vi "定时触发器.vi"(9 "绝对定时忽略0帧? (T)":bool=TRUE, 10 "定时配置":T1={"定时模式"=enum."绝对时间", "单位"=enum."年", "间隔"=1, "目标时刻"=timestamp(0 s since 1904-01-01)} {"间隔" min=1}, 11 "定时器结构名":string="L229074972") -> ()   [LabVIEW 2017]
doc: "可重入的定时触发源, 相对定时和绝对定时. \n\n绝对定时 在运行启动或重新配置之后,可按需求设定是否忽略0帧触发;\n相对定时 在运行启动时重新配置之后,强制执行0帧触发."
uses:
  <vilib>/Platform/TimedLoop/XDataNode/timing_clust.ctl
  <vilib>/Platform/TimedLoop/XDataNode/nitl_modes.ctl
  <vilib>/Platform/TimedLoop/XDataNode/wakeup.ctl
  <vilib>/Platform/TimedLoop/XDataNode/XDataNode.xnode
  <vilib>/Platform/TimedLoop/XDataNode/XDNodeRunTimeDep.lvlib
panel:
  in  "重启定时":bool
  in  "结构名":string="L229074972"
  out "上次触发":timestamp
  # "用法:\n1. 使用异步调用\n2. 改变输入, 调用定时结构停止函数, 实现重启并应用新的定时配置\n\n注意:\n此VI中, 首次启动或重新配置定时循环时不触发值改变事件"
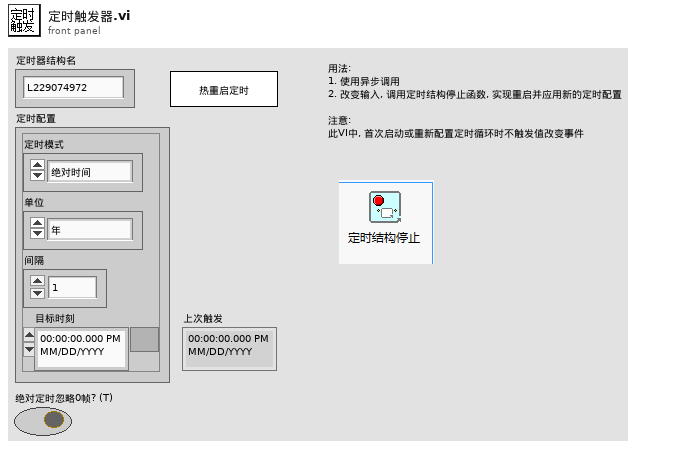
[diagram p1: front panel]
types:
  T1 = typedef "簇-定时配置.ctl" = cluster{"定时模式":enum16{"绝对时间", "相对时间"}, "单位":enum16{"年", "月", "日", "时", "分"}, "间隔":u8, "目标时刻":timestamp}
  T2 = typedef "XDNodeRunTimeDep.lvlib/timing_clust.ctl" = cluster{"Expected End [f-1]":u64, "Actual End [f-1]":u64, "Finished Late? [f-1]":bool, "Expected End [i-1]":u64, "Actual End [i-1]":u64, "Finished Late? [i-1]":bool, "Expected Start [i]":u64, "Actual Start [i]":u64, "Expected Start [f]":u64, "Actual Start [f]":u64, "Source Name":string, "Structure Name":string, "Period":i64, "Deadline":i64, "Offset":i64, "Start":i64, "Priority":i32, "Timeout":i32, "Mode":T3, "Wakeup Reason":T4, "Error":errorcluster, "Source Type":string, "Secondary Source Type":string, "Global End Time":u64, "Global Start Time":u64, "Frame Duration":u64, "Iteration Duration":u64, "Assigned CPU":i32, "I/O Scan Engine Mode":u32}
  T3 = typedef "XDNodeRunTimeDep.lvlib/nitl_modes.ctl" = enum32{"No Change", "Process missed periods, maintain original phase", "Discard missed periods, maintain original phase", "Process missed periods, ignore original phase", "Discard missed periods, ignore original phase"}
  T4 = typedef "XDNodeRunTimeDep.lvlib/wakeup.ctl" = enum32{"Normal", "Aborted", "Asynchronous wakeup", "Timing source error", "Timed loop error", "Timeout"}
  T5 = typedef "LVDateTimeRec.ctl" = cluster{"秒数的小数部分":dbl, "秒":i32, "分":i32, "时":i32, "日":i32, "月":i32, "年":i32, "天数（周）":i32, "天数（年）":i32, "DST":i32}
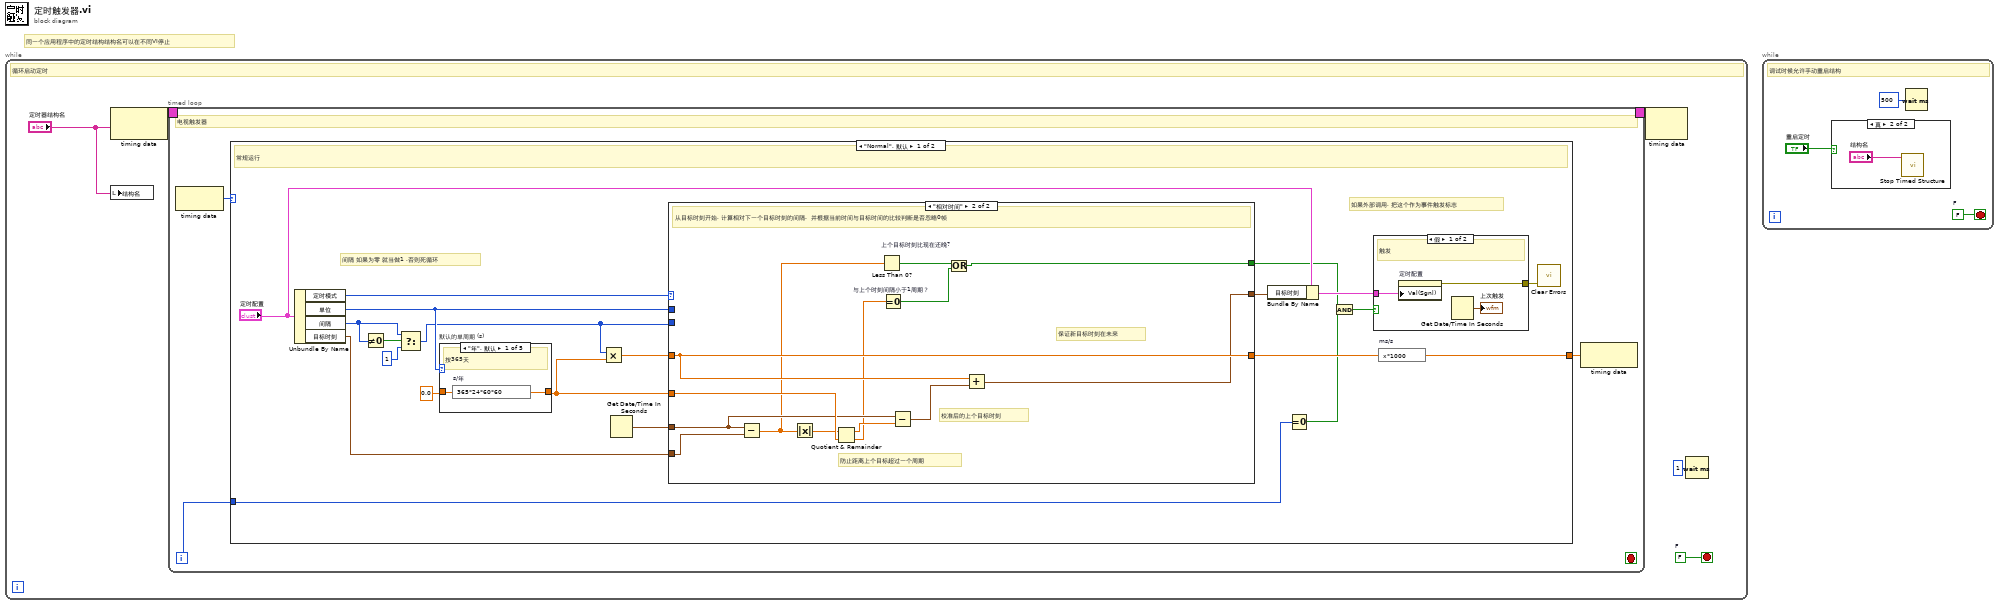
[diagram p0: block diagram]
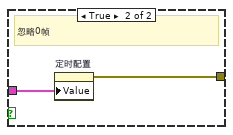
[diagram p3: hidden frame]
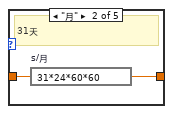
[diagram p4: hidden frame]
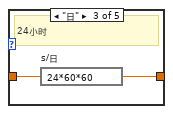
[diagram p5: hidden frame]
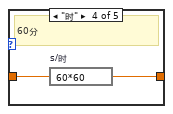
[diagram p6: hidden frame]
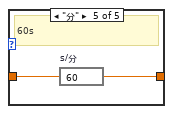
[diagram p7: hidden frame]
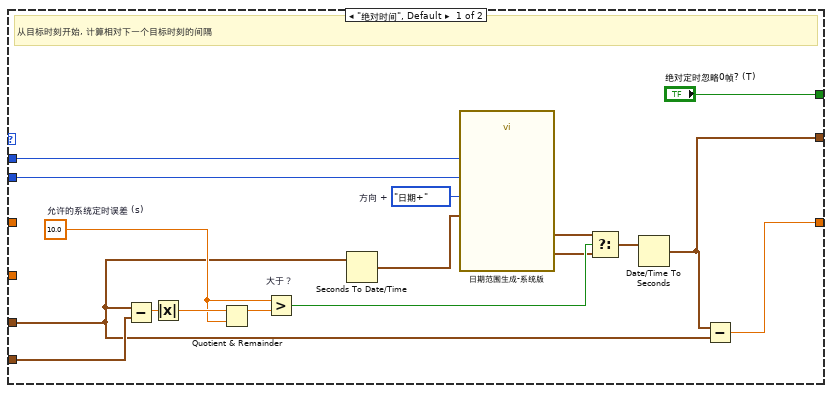
[diagram p8: hidden frame]
diagram:
  # "同一个应用程序中的定时结构结构名可以在不同VI停止"
  n1 = while {
    stop <- w3 stop-if-true
    w3 = FALSE  # F
    # "循环启动定时"
    n2 = node-c288("定时器结构名") -> (w5:T2)
    n3 = local write "结构名"("定时器结构名") -> ()
    n4 = timed-loop {
      timing: w5 -> [_]
      timing-out: [_] -> w4
      i -> [w7]
      stop <- _ stop-if-true
      # "电视触发器"
      n5 = node-c288() -> (w6:T4)  [unwired: 1 in]
      n6 = case shown="\"Normal\", 默认" w6 {
        tunnel: [w25 _] -> w8
        tunnel: w7 -> [w15 _]
        frame "Normal", Default {
          # "间隔 如果为零 就当做1 ,否则死循环"
          # "如果外部调用, 把这个作为事件触发标志"
          # "常规运行"
          n7 = Unbundle By Name("定时配置") -> ("定时模式"=w29:enum16{"绝对时间", "相对时间"}, "单位"=w28:enum16{"年", "月", "日", "时", "分"}, "间隔"=w17:u8, "目标时刻"=w24:timestamp)
          n8 = Not Equal To 0?(x=w17) -> (x != 0?=w19:bool)
          n9 = Select(t=w17, s=w19, f=u8 1 ("间隔")) -> (s? t:f=w16:u8)
          n10 = case "默认的单周期 (s)" shown="\"年\", 默认" w28 {
            tunnel: [w36 w38 w40 w42 w44] -> w9
            tunnel: 0.0 -> [w35 w37 w39 w41 w43]
            frame "年", Default {
              # "按365天"
              n11 = expression code="365*24*60*60" "s/年"(w35) -> (w36:dbl)
            }
            frame "月" {
              # "31天"
              n12 = expression code="31*24*60*60" "s/月"(w37) -> (w38:dbl)
            }
            frame "日" {
              # "24小时"
              n13 = expression code="24*60*60" "s/日"(w39) -> (w40:dbl)
            }
            frame "时" {
              # "60分"
              n14 = expression code="60*60" "s/时"(w41) -> (w42:dbl)
            }
            frame "分" {
              # "60s"
              n15 = expression code="60" "s/分"(w43) -> (w44:dbl)
            }
          }
          n16 = Multiply(x=w16, y=w9) -> (x*y=w23:dbl)
          n17 = Get Date/Time In Seconds() -> (seconds since 1Jan1904=w10:timestamp)
          n18 = case shown="\"相对时间\"" w29 {
            tunnel: w28 -> [w61 _]
            tunnel: w16 -> [w56 _]
            tunnel: [w59 w74] -> w26
            tunnel: w24 -> [w57 w69]
            tunnel: w23 -> [_ w74]
            tunnel: [w55 w73] -> w20
            tunnel: ["绝对定时忽略0帧? (T)" w64] -> w11
            tunnel: w10 -> [w45 w71]
            tunnel: w9 -> [_ w72]
            frame "绝对时间", Default {
              w47 = 10.0  # 允许的系统定时误差 (s)
              w54 = enum16{"当前", "日期+", "日期-"}."日期+"  # 方向 +
              # "从目标时刻开始, 计算相对下一个目标时刻的间隔"
              n19 = Subtract(x=w45, y=w57) -> (x-y=w58:dbl)
              n20 = Absolute Value(x=w58) -> (abs(x)=w49:dbl)
              n21 = Quotient & Remainder(x=w49, y=w47) -> (x-y*floor(x/y)=w48:dbl)  [unwired: 1 out]
              n22 = Greater? "大于？"(x=w47, y=w48) -> (0:w53:bool)
              n23 = Seconds To Date/Time(time stamp (now)=w45) -> (date time rec=w60:T5)  [unwired: 1 in]
              n24 = call "日期范围生成-系统版.vi"("单位"=w61, "方向"=w54, "变化量(1)"=w56, "日期时间记录"=w60) -> ("下限"=w51:T5, "上限"=w50:T5)  [unwired: 6 in]
              n25 = Select(t=w51, s=w53, f=w50) -> (s? t:f=w52:T5)
              n26 = Date/Time To Seconds(2:w52) -> (0:w55:timestamp)  [unwired: 1 in]
              n27 = Subtract(x=w55, y=w45) -> (x-y=w59:dbl)
            }
            frame "相对时间" {
              # "保证新目标时刻在未来"
              # "校准后的上个目标时刻"
              # "防止距离上个目标超过一个周期"
              # "从目标时刻开始, 计算相对下一个目标时刻的间隔.  并根据当前时间与目标时间的比较判断是否忽略0帧"
              n28 = Subtract(x=w71, y=w69) -> (x-y=w66:dbl)
              n29 = Absolute Value(x=w66) -> (abs(x)=w67:dbl)
              n30 = Quotient & Remainder(x=w67, y=w72) -> (x-y*floor(x/y)=w70:dbl, floor(x/y)=w63:dbl)
              n31 = Less Than 0? "上个目标时刻比现在还晚?"(x=w66) -> (x < 0?=w65:bool)
              n32 = Equal To 0? "与上个时刻间隔小于1周期？"(x=w63) -> (x = 0?=w62:bool)
              n33 = Subtract(x=w71, y=w70) -> (x-y=w68:timestamp)
              n34 = Or(x=w65, y=w62) -> (x .or. y?=w64:bool)
              n35 = Add(x=w74, y=w68) -> (x+y=w73:timestamp)
            }
          }
          n36 = Bundle By Name(cluster="定时配置", "目标时刻"=w20) -> (w21:T1)
          n37 = Equal To 0?(x=w15) -> (x = 0?=w14:bool)
          n38 = And(x=w11, y=w14) -> (x .and. y?=w13:bool)
          n39 = case shown="假" w13 {
            tunnel: w21 -> [w32 w34]
            tunnel: [w31 w33] -> w12
            frame False {
              # "触发"
              n40 = property on="定时配置" class="Clust (严格)"("Val(Sgnl)"=w32) -> (error out=w31:errorcluster)  [unwired: 2 in, 1 out]
              n41 = Get Date/Time In Seconds() -> (seconds since 1Jan1904=→"上次触发":timestamp)
            }
            frame True {
              # "忽略0帧"
              n42 = property on="定时配置" class="Clust (严格)"("Value"=w34) -> (error out=w33:errorcluster)  [unwired: 2 in, 1 out]
            }
          }
          n43 = expression code="x*1000" "ms/s"(w26) -> (w25:dbl)
          n44 = call <vilib>:"Clear Errors.vi"("error in (no error)"=w12) -> ()  [unwired: 5 in, 2 out]
        }
        frame "Aborted" {
          # "外部终止了此定时循环结构"
        }
      }
      n45 = node-c288(w8) -> ()  [unwired: 1 out]
    }
    n46 = node-c288(w4) -> ()  [unwired: 1 out]
    n47 = Wait (ms)(milliseconds to wait=u32 1 ("等待时间（毫秒）")) -> ()  [unwired: 1 out]
  }
  n48 = while {
    stop <- w86 stop-if-true
    w86 = FALSE  # F
    # "调试时候允许手动重启结构"
    n49 = case shown="真" "重启定时" {
      frame False {
      }
      frame True {
        n50 = call <vilib>:"Stop Timed Structure.vi"("name"="结构名") -> ()  [unwired: 10 in, 1 out]
      }
    }
    n51 = Wait (ms)(milliseconds to wait=u32 500 ("等待时间（毫秒）")) -> ()  [unwired: 1 out]
  }
